vi "Measurement Logic.vi"(8 "error in":errorcluster, 11 "Measurement Configuration":T2) -> (0 "error out":errorcluster, 3 "Measurement Results":T1)   [LabVIEW 2020, in "MeasurementService_Template.lvlib"]
uses:
  MeasurementService_Template.lvlib
  Measurement Configuration.ctl
  Measurement Results.ctl
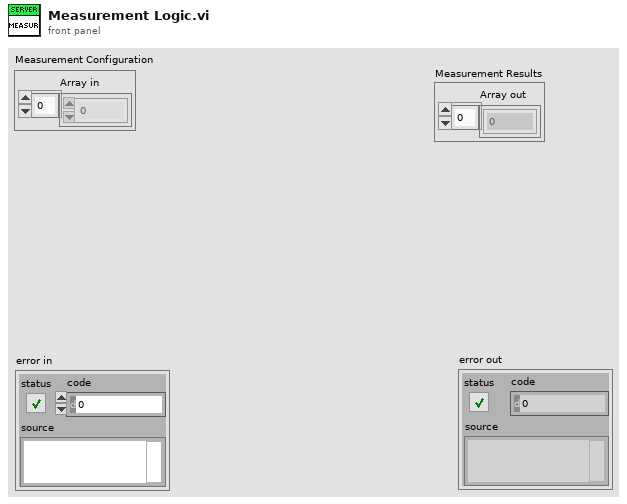
[diagram p1: front panel]
types:
  T1 = typedef "MeasurementService_Template.lvlib/Measurement Results.ctl" = cluster{"Array out":dbl[]}
  T2 = typedef "MeasurementService_Template.lvlib/Measurement Configuration.ctl" = cluster{"Array in":dbl[]}
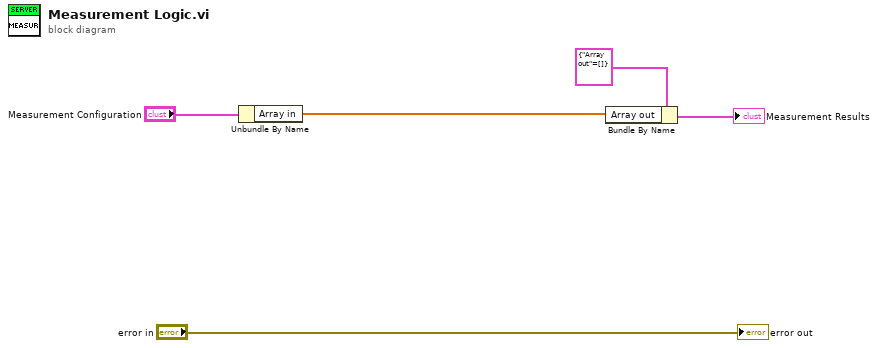
[diagram p0: block diagram]
diagram:
  n1 = Unbundle By Name("Measurement Configuration") -> ("Array in"=w1:dbl[])
  n2 = Bundle By Name(cluster=T1 {"Array out"=[]} ("Measurement Results"), "Array out"=w1) -> (→"Measurement Results":T1)
  "error out" <- "error in"
